vi "SA_Save_File_SubVI.vi"(7 "spreadsheet string":string, 8 "error in (no error)":errorcluster, 9 "string":string, 10 "Base Name":string, 11 "file (use dialog)":path) -> (0 "error out":errorcluster)   [LabVIEW 2023, in "SpectrumAnalyzerUI.lvlib" / "SpectrumAnalyzerUI.lvclass"]
uses:
  SpectrumAnalyzerUI.lvclass
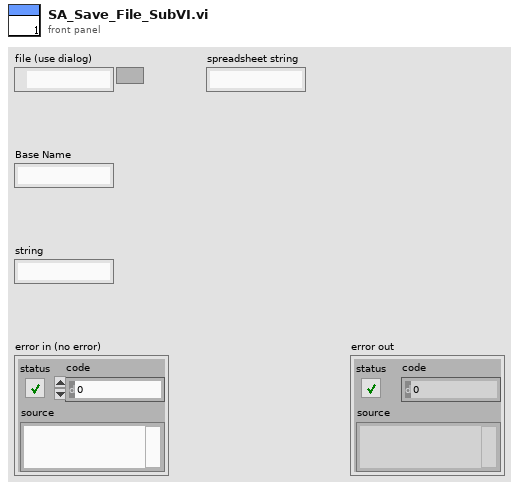
[diagram p1: front panel]
types:
  T1 = enum16{"open", "replace", "create", "open or create", "replace or create", "replace or create with confirmation"}
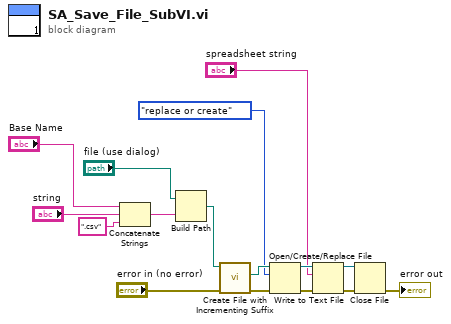
[diagram p0: block diagram]
diagram:
  n1 = Concatenate Strings("Base Name", "string", ".csv" ("string")) -> (w2:string)
  n2 = Build Path(base path="file (use dialog)", name or relative path=w2) -> (appended path=w10:path)
  n3 = call <vilib>:"Create File with Incrementing Suffix.vi"("error in (no error)"="error in (no error)", "file path"=w10) -> ("error out"=w14:errorcluster, "actual path"=w12:path)  [unwired: 7 in, 1 out]
  n4 = Open/Create/Replace File(file path (use dialog)=w12, error in=w14, operation (0:open)=T1."replace or create") -> (refnum out=w16:refnum<file>, error out=w15:errorcluster)  [unwired: 3 in, 1 out]
  n5 = Write to Text File(file (use dialog)=w16, text="spreadsheet string", error in=w15) -> (refnum out=w7:refnum<file>, error out=w8:errorcluster)  [unwired: 1 in, 1 out]
  n6 = Close File(refnum=w7, error in=w8) -> (error out=→"error out":errorcluster)  [unwired: 1 out]
